vi "get_cuda_available_devices.vi"(8 "Error in":errorcluster caption="Error in (no error)") -> (0 "Error out":errorcluster, 1 "error_code":i32, 3 "num_cuda_devices":i32)   [LabVIEW 2018]
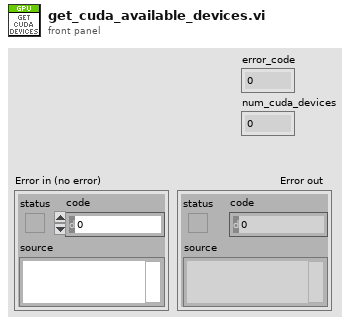
[diagram p1: front panel]
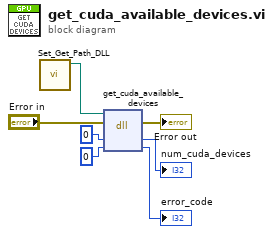
[diagram p0: block diagram]
diagram:
  n1 = call "Set_Get_Path_DLL.vi"() -> ("path DLL Out"=w1:path)  [unwired: 11 in]
  n2 = dll-call lib="C:/Users/AUTIS/Documents/TFG/Proyecto/LabVIEW_PRUEBAS/VIs/Utilidades/DLL/SR_GPU_TOOLKIT.dll" fn="get_cuda_available_devices"(path in=w1, error in="Error in", "num_cuda_devices"=0, "error_code"=0) -> (error out=→"Error out":errorcluster, "num_cuda_devices"=→"num_cuda_devices":i32, "error_code"=→"error_code":i32)  [unwired: 2 in, 1 out]
